vi "Temperature controller Front Panel.vi"(8 "error in (no error)":errorcluster, 11 "Class":refnum<class "Temperature controller.lvclass">) -> (0 "error out":errorcluster, 3 "Temperature controller out":refnum<class "Temperature controller.lvclass">)   [LabVIEW 2015]
uses:
  Temperature controller.lvclass
panel:
  in  "Measure heater":bool
  in  "Measure R":bool
  in  "Channels to measure":i32[](array[numeric])=[1]
  # "(CH A=1)"
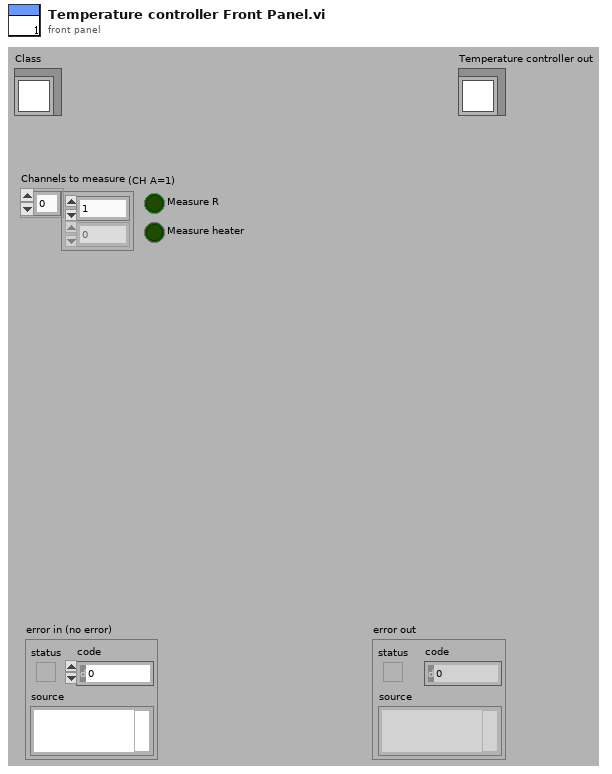
[diagram p1: front panel]
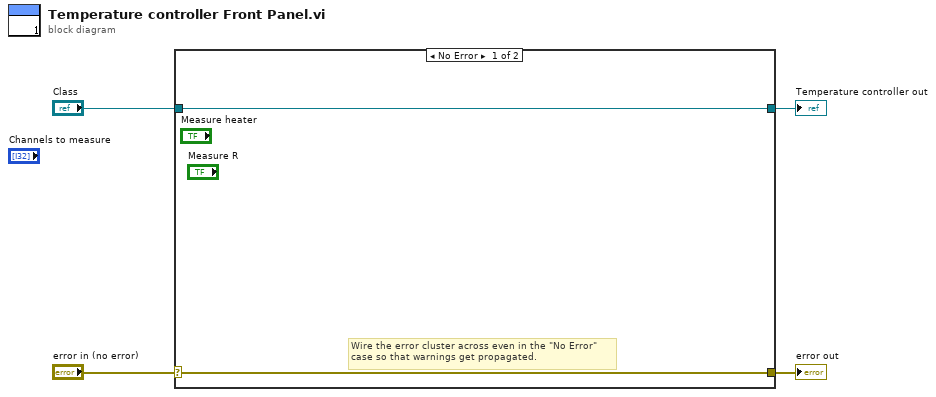
[diagram p0: block diagram]
diagram:
  n1 = case shown="No Error" "error in (no error)" {
    selector: "error in (no error)" -> [w5 w8]
    tunnel: [w5 w8] -> w3
    tunnel: [w6 w7] -> w1
    tunnel: "Class" -> [w6 w7]
    frame No Error {
      # "Wire the error cluster across even in the \"No Error\"\ncase so that warnings get propagated."
    }
    frame Error {
    }
  }
  "error out" <- w3
  "Temperature controller out" <- w1
